vi "生成一个在一米到两米之间的随机长度.vi"() -> ()   [LabVIEW 2020]
uses:
  <vilib>/numeric/Random Number (Range) DBL.vi
panel:
  out "数值":dbl[unit]
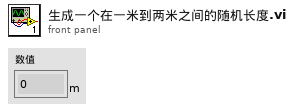
[diagram p1: front panel]
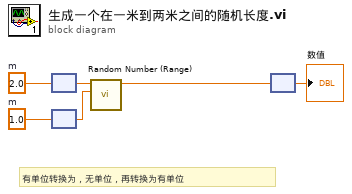
[diagram p0: block diagram]
diagram:
  w6 = dbl[unit] 1.0  # m
  w3 = dbl[unit] 2.0  # m
  # "有单位转换为，无单位，再转换为有单位"
  n1 = node(w3) -> (w4:dbl)
  n2 = node(w6) -> (w5:dbl)
  n3 = call-poly <vilib>:"Random Number (Range).vi"("lower bound (0)"=w5, "upper bound (100)"=w4) -> ("number"=w2:dbl)  [unwired: 9 in]
  n4 = node(w2) -> (→"数值":dbl[unit])
